vi "JPL Array.vi"(10 "Boolean 2":bool, 11 "Boolean":bool) -> (2 "Value":dbl, 3 "Index":dbl)   [LabVIEW 2015]
uses:
  <vilib>/functionblocks/Edge Detection/One Shot Rising with Input/One Shot Rising with Input.vi
  <vilib>/functionblocks/FB Core/FB Core.xnode
  <vilib>/functionblocks/NI_FunctionBlock Libraries.lvlib
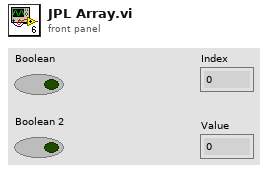
[diagram p1: front panel]
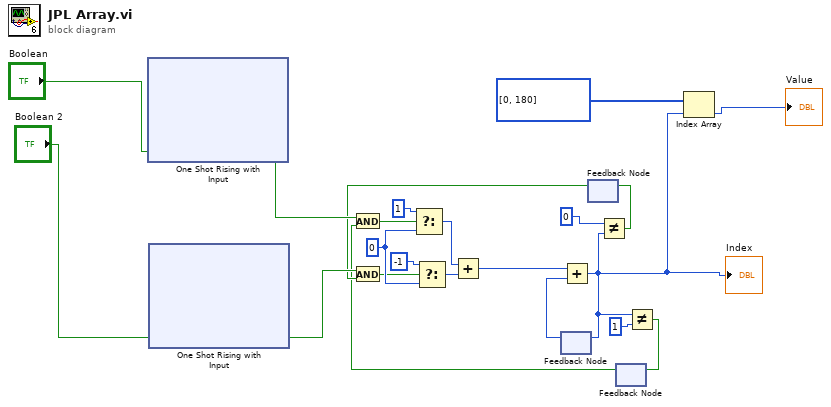
[diagram p0: block diagram]
diagram:
  w12 = 0
  n1 = xnode "One Shot Rising with Input"("input"="Boolean") -> ("output"=w21:bool)  [unwired: 1 in, 1 out]
  n2 = xnode "One Shot Rising with Input"("input"="Boolean 2") -> ("output"=w22:bool)  [unwired: 1 in, 1 out]
  n3 = feedback #1() -> (w20:i32)  [unwired: 1 in]
  n4 = feedback #2() -> (w5:bool)  [unwired: 1 in]
  n5 = And(x=w22, y=w5) -> (x .and. y?=w8:bool)
  n6 = Select(t=-1, s=w8, f=w12) -> (s? t:f=w14:i32)
  n7 = feedback #3() -> (w3:bool)  [unwired: 1 in]
  n8 = And(x=w21, y=w3) -> (x .and. y?=w9:bool)
  n9 = Select(t=1, s=w9, f=w12) -> (s? t:f=w13:i32)
  n10 = Add(x=w13, y=w14) -> (x+y=w15:i32)
  n11 = Add(x=w15, y=w20) -> (x+y=w18:i32)
  "Index" <- w18
  n12 = feedback-in #1(w18) -> ()
  n13 = Not Equal?(x=0, y=w18) -> (x != y?=w6:bool)
  n14 = feedback-in #2(w6) -> ()
  n15 = Not Equal?(x=w18, y=1) -> (x != y?=w4:bool)
  n16 = feedback-in #3(w4) -> ()
  n17 = Index Array(array=i32[] [0, 180], index=w18) -> (element=→"Value":i32)
